vi "UTIL Hourly File Path.vi"(8 "Error In":errorcluster, 10 "Testing":bool) -> (0 "Error Out":errorcluster, 3 "Hourly File Path":path)   [LabVIEW 2010]
doc: "Given a Data Folder, this creates a File Path of the form <Folder>\\Raw Data_mmddHH.bin, where mmddHH are 2-digit month, 2-digit day, 2-digit 24-hour numbers. The first time this is called, the file name corresponds to the current date/time. On subsequent calls, it uses the same name unless at least an hour has passed, in which case it creates a new filename using the same format.\n\nInputs:\n Data Folder Path to a Folder\n Error In\nOutputs:\n Hourly File Path Path of the form <Data Folder>\\Raw Data_mmddHH.bin\n Error Out"
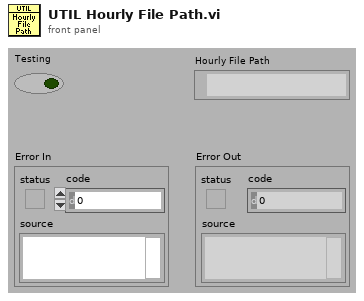
[diagram p1: front panel]
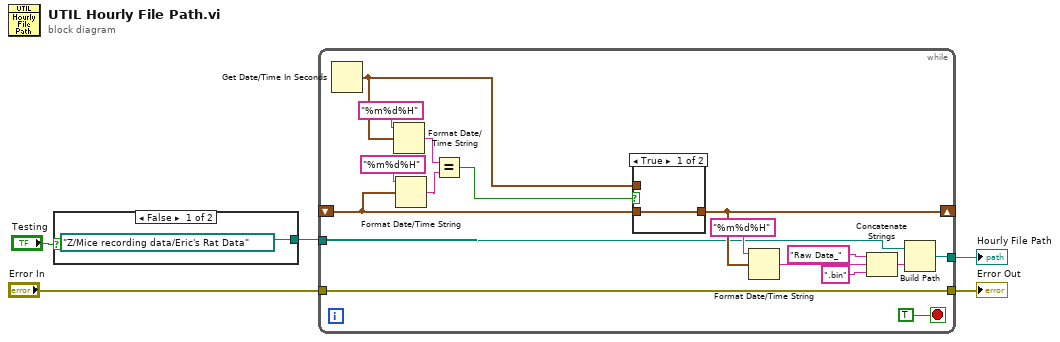
[diagram p0: block diagram]
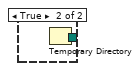
[diagram p2: hidden frame]
diagram:
  n1 = case shown="False" "Testing" {
    tunnel: [path "Z:/Mice recording data/Eric's Rat Data" ("base path") w7] -> w1
    frame False {
    }
    frame True {
      n2 = Temporary Directory() -> (w7:path)
    }
  }
  n3 = while {
    tunnel: "Error In" -> [w22]
    shift-right: [w24] -> _
    shift-left: _ -> [w9]
    tunnel: [w22] -> w4
    tunnel: [w17] -> w3
    tunnel: w1 -> [w15]
    stop <- TRUE stop-if-true
    n4 = Get Date/Time In Seconds() -> (seconds since 1Jan1904=w13:timestamp)
    n5 = Format Date/Time String(time format string (%c)="%m%d%H", seconds (now)=w13) -> (date/time string=w12:string)  [unwired: 1 in]
    n6 = Format Date/Time String(time format string (%c)="%m%d%H", seconds (now)=w9) -> (date/time string=w8:string)  [unwired: 1 in]
    n7 = Equal?(x=w12, y=w8) -> (x = y?=w11:bool)
    n8 = case shown="True" w11 {
      tunnel: w13 -> [_ w26]
      tunnel: [w25 w26] -> w24
      tunnel: w9 -> [w25 _]
      frame True {
      }
      frame False {
      }
    }
    n9 = Format Date/Time String(time format string (%c)="%m%d%H", seconds (now)=w24) -> (date/time string=w21:string)  [unwired: 1 in]
    n10 = Concatenate Strings("Raw Data_" ("string"), w21, ".bin" ("string")) -> (w18:string)
    n11 = Build Path(base path=w15, name or relative path=w18) -> (appended path=w17:path)
  }
  "Error Out" <- w4
  "Hourly File Path" <- w3
